vi "2_7.vi"() -> ()   [LabVIEW 2015]
panel:
  in  "Replace String":string
  in  "Search String":string
  out "Result String":string
  in  "String":string
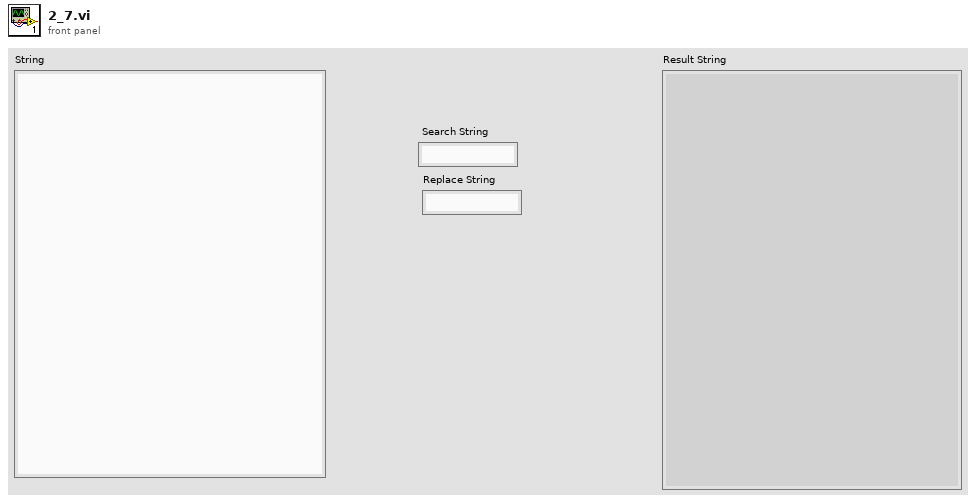
[diagram p1: front panel]
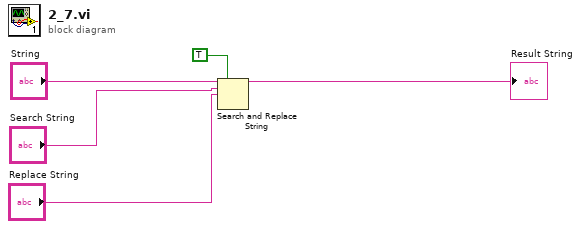
[diagram p0: block diagram]
diagram:
  n1 = Search and Replace String(replace all?=TRUE ("replace all? (F)"), input string="String", search string="Search String", replace string="Replace String") -> (result string=→"Result String":string)  [unwired: 4 in, 3 out]
